vi "Flush Specific.vi"(7 "Q Ref In":refnum<queue>, 8 "error in":errorcluster, 11 "Messages to Remove":string[](array[string])) -> (0 "error out":errorcluster, 5 "Q Ref Out":refnum<queue>)   [LabVIEW 2025, in "Q Wrappers.lvlib"]
uses:
  Q Wrappers.lvlib
  Q Packet.ctl
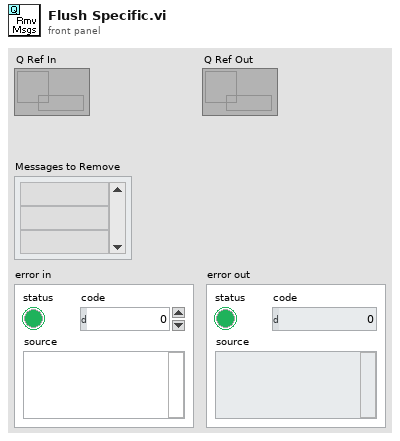
[diagram p1: front panel]
types:
  T1 = typedef "Q Packet.ctl" = cluster{"Message ID":string, "Payload":variant}
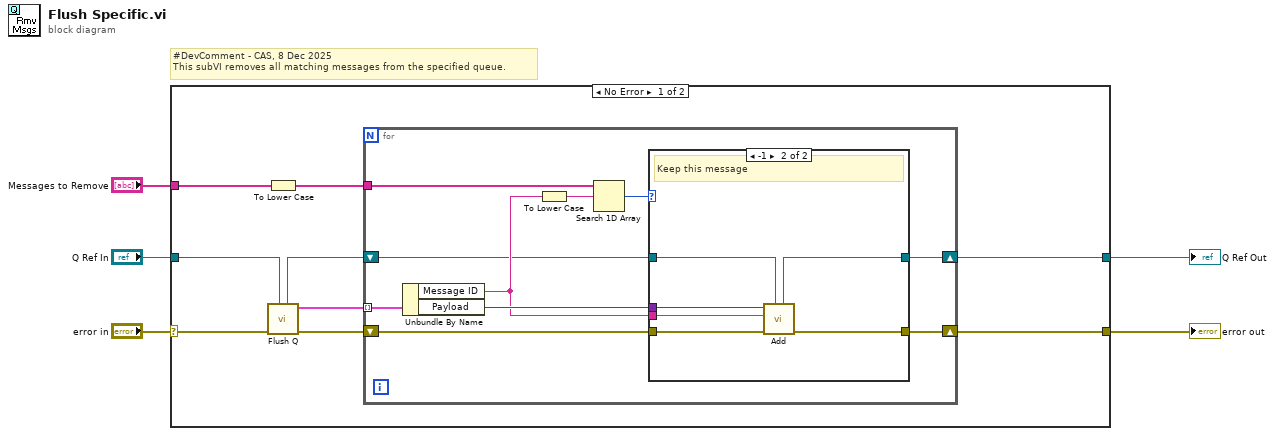
[diagram p0: block diagram]
diagram:
  # "#DevComment - CAS, 8 Dec 2025\nThis subVI removes all matching messages from the specified queue."
  n1 = case shown="No Error" "error in" {
    selector: "error in" -> [w12 w34]
    tunnel: [w14 w34] -> w4
    tunnel: "Q Ref In" -> [w9 w33]
    tunnel: "Messages to Remove" -> [w13 _]
    tunnel: [w6 w33] -> w1
    frame No Error {
      n2 = To Lower Case(string=w13) -> (all lower case string=w7:string[])
      n3 = call "Flush Q.vi"("Q Ref In"=w9, "error in"=w12) -> ("error out"=w11:errorcluster, "Remaining Elements"=w8:T1[], "Q Ref Out"=w10:refnum<queue>)  [unwired: 7 in]
      n4 = for {
        shift-right: [w23] -> w14
        shift-left: w11 -> [w24]
        tunnel: w7 -> [w21]
        tunnel: w8 -> [w20] mode=indexing
        shift-right: [w15] -> w6
        shift-left: w10 -> [w16]
        n5 = Unbundle By Name(w20) -> ("Message ID"=w17:string, "Payload"=w19:variant)
        n6 = To Lower Case(string=w17) -> (all lower case string=w18:string)
        n7 = Search 1D Array(1D array=w21, element=w18) -> (index of element=w22:i32)  [unwired: 1 in]
        n8 = case shown="-1" w22 {
          tunnel: w24 -> [w26 w32]
          tunnel: [w26 w31] -> w23
          tunnel: w19 -> [_ w30]
          tunnel: w17 -> [_ w29]
          tunnel: w16 -> [w25 w28]
          tunnel: [w25 w27] -> w15
          frame Default {
            # "Remove this message"
          }
          frame -1 {
            # "Keep this message"
            n9 = call "Add.vi"("Q Ref In"=w28, "error in"=w32, "Message ID"=w29, "Payload"=w30) -> ("error out"=w31:errorcluster, "Q Ref Out"=w27:refnum<queue>)  [unwired: 4 in, 2 out]
          }
        }
      }
    }
    frame Error {
    }
  }
  "error out" <- w4
  "Q Ref Out" <- w1
